vi "Get Public API.vi"(8 "error in (no error)":errorcluster, 11 "VNA":refnum<class "VNA.lvclass">) -> (0 "error out":errorcluster, 2 "Commands":string[](array[string]), 3 "VNA out":refnum<class "VNA.lvclass">)   [LabVIEW 2016, in "VNA.lvclass"]
uses:
  VNA.lvclass
  Typedefs/VNA.Commands.ctl
  <userlib>/LevyLab/Levylab Instruments/Instrument Types/VNA/Instrument.VNA.lvclass
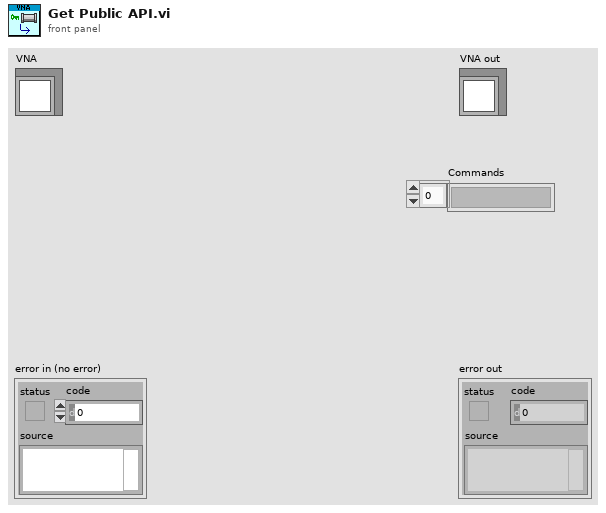
[diagram p1: front panel]
types:
  T1 = typedef "VNA.lvclass/VNA.Commands.ctl" = string[]
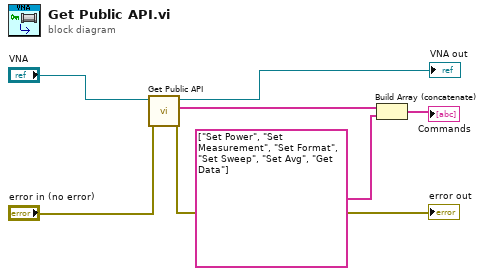
[diagram p0: block diagram]
diagram:
  n1 = call-parent "Get Public API.vi"("error in (no error)"="error in (no error)", "Instrument in"="VNA") -> ("error out"=→"error out":errorcluster, "Commands"=w6:string[], "Instrument out"=→"VNA out":refnum<class "VNA.lvclass">)  [unwired: 7 in]
  n2 = Build Array (concatenate)(w6, T1 ["Set Power", "Set Measurement", "Set Format", "Set Sweep", "Set Avg", "Get Data"] ("Array")) -> (→"Commands":T1)
